vi "Blackout.vi"(10 "Drawing Mode (Frame)":u32(ring) items=["Frame", "Fill", "Highlight"], 11 "Image":T1) -> (3 "Image Out":T1)   [LabVIEW 2012]
uses:
  <vilib>/vision/Image Controls.llb/IMAQ Image.ctl
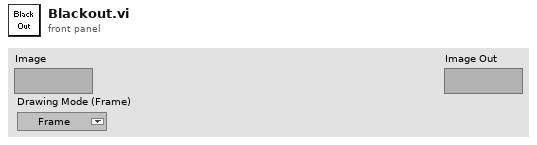
[diagram p1: front panel]
types:
  T1 = typedef "IMAQ Image.ctl" = refnum<image>
  T2 = cluster{"Left":i32, "Top":i32, "Right":i32, "Bottom":i32}
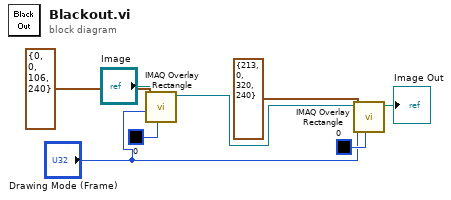
[diagram p0: block diagram]
diagram:
  n1 = call "IMAQ Overlay Rectangle"("Color"=u32 0, "Drawing Mode (Frame)"="Drawing Mode (Frame)", "Rectangle"=T2 {"Left"=0, "Top"=0, "Right"=106, "Bottom"=240}, "Image"="Image") -> ("Image Out"=w8:T1)  [unwired: 2 in, 5 out]
  n2 = call "IMAQ Overlay Rectangle"("Color"=u32 0, "Drawing Mode (Frame)"="Drawing Mode (Frame)", "Rectangle"=T2 {"Left"=213, "Top"=0, "Right"=320, "Bottom"=240}, "Image"=w8) -> ("Image Out"=→"Image Out":T1)  [unwired: 2 in, 5 out]
